vi "Version_2.0_Single_Column_Code.vi"() -> ()   [LabVIEW 2020] (continued)
                                n1984 = Subtract(x=w2419, y=w2420) -> (x-y=w2418:dbl)
                                n1985 = Absolute Value(x=w2418) -> (abs(x)=w2417:dbl)
                                }
                                frame "High Resolution Pumping" {
                                n1986 = local read "Buffer-C2 Volume \nto be Pumped"() -> (w2431:dbl)
                                n1987 = local read "Volume of Syringe"() -> (w2434:dbl)
                                n1988 = local read "Initial Plunger Position"() -> (w2438:dbl)
                                n1989 = local read "Position\nNow"() -> (w2437:dbl)
                                n1990 = Subtract(x=w2438, y=w2437) -> (x-y=w2436:dbl)
                                n1991 = Absolute Value(x=w2436) -> (abs(x)=w2435:dbl)
                                n1992 = Multiply(x=w2435, y=w2434) -> (x*y=w2433:dbl)
                                n1993 = Divide(x=w2433, y=24000.0) -> (x/y=w2430:dbl)
                                n1994 = Subtract(x=w2430, y=w2431) -> (x-y=w2429:dbl)
                                n1995 = Absolute Value(x=w2429) -> (abs(x)=w2428:dbl)
                                }
                                }
                                n1996 = local write "Buffer-C Volume\nleft to be Pumped"(w2415) -> ()
                                }
                                frame #2 {
                                n1997 = local read "Buffer-C2 Dispense\nFlow Rate (ul/min)"() -> (w2442:dbl)
                                n1998 = local read "Buffer-C2 Pumping\nResolution"() -> (w2441:T2)
                                n1999 = local read "VISA Refnum in\nfor Pump"() -> (w2444:refnum<visa-resource-name>)
                                n2000 = local read "Volume of Syringe"() -> (w2443:dbl)
                                n2001 = call "GoToAbsolutePosition(SubVI).vi"("Absolute Volume Position in Syringe (in ul)"=0.0, "Volume of Syringe"=w2443, "Resolution of Pumping"=w2441, "Flow Rate (ul/min)"=w2442, "VISA Refnum in"=w2444) -> ()  [unwired: 6 in, 1 out]
                                n2002 = local write "Suction On/Off"(FALSE ("Suction On/Off")) -> ()
                                }
                                }
                                }
                                }
                                }
                                frame #4 {
                                n2003 = local read "Stop for End of \nExperiment \nand Data Writing"() -> (w2445:bool)
                                n2004 = case shown="True" w2445 {
                                frame False {
                                }
                                frame True {
                                n2005 = local read "VISA Refnum in\nfor Pump"() -> (w2446:refnum<visa-resource-name>)
                                n2006 = call "HardStopCurrentProcess (SubVI).vi"("VISA Refnum in"=w2446) -> ()  [unwired: 11 in]
                                }
                                }
                                }
                                }
                                }
                                frame #2 {
                                # "Keeps the on-chip valve V1, V2 Open and V3 closed"
                                n2007 = while {
                                stop <- w2450 stop-if-true
                                n2008 = local read "Suction On/Off"() -> (w2451:bool)
                                n2009 = case shown="True" w2451 {
                                frame False {
                                n2010 = local read "Buffer-C2 Pumping\nResolution"() -> (w2457:T2)
                                n2011 = local read "Initial Plunger Position"() -> (w2456:dbl)
                                n2012 = local read "VISA Refnum in\nfor Pump"() -> (w2458:refnum<visa-resource-name>)
                                n2013 = local read "Position\nNow"() -> (w2454:dbl)
                                n2014 = local read "Volume of Syringe"() -> (w2455:dbl)
                                n2015 = local write "Volume being Injected \nin this process"(0.0) -> ()
                                n2016 = local write "Pause Data Collection"(FALSE) -> ()
                                n2017 = while {
                                tunnel: w2458 -> [w2465]
                                tunnel: w2457 -> [w2464]
                                tunnel: w2456 -> [w2460]
                                tunnel: w2455 -> [w2463]
                                tunnel: w2454 -> [w2459]
                                stop <- w2461 stop-if-true
                                n2018 = stacked-sequence {
                                tunnel: w2465 -> [w2471 w2493 w2518]
                                tunnel: w2464 -> [w2470 w2492 _]
                                tunnel: w2460 -> [w2468 _ _]
                                tunnel: w2463 -> [w2467 w2490 _]
                                tunnel: [_ _ w2510] -> w2461
                                tunnel: w2459 -> [_ w2488 _]
                                frame #0 {
                                # "From here on 'True Volume being injected \nin this process' represents the true total \nvolume in this process"
                                n2019 = call "AbsolutePlungerPosition (SubVI).vi"("VISA Refnum in"=w2471) -> ("Plunger Position"=w2469:i32)  [unwired: 10 in]
                                n2020 = case shown="..\"Standard Pumping\"" w2470 {
                                tunnel: w2469 -> [w2479 w2487]
                                tunnel: w2468 -> [w2478 w2486]
                                tunnel: w2467 -> [w2475 w2483]
                                tunnel: [w2472 w2480] -> w2466
                                frame .."Standard Pumping" {
                                n2021 = Subtract(x=w2479, y=w2478) -> (x-y=w2477:dbl)
                                n2022 = Absolute Value(x=w2477) -> (abs(x)=w2476:dbl)
                                n2023 = Multiply(x=w2476, y=w2475) -> (x*y=w2474:dbl)
                                n2024 = Divide(x=w2474, y=3000.0) -> (x/y=w2472:dbl)
                                }
                                frame "High Resolution Pumping".. {
                                n2025 = Subtract(x=w2487, y=w2486) -> (x-y=w2485:dbl)
                                n2026 = Absolute Value(x=w2485) -> (abs(x)=w2484:dbl)
                                n2027 = Multiply(x=w2484, y=w2483) -> (x*y=w2482:dbl)
                                n2028 = Divide(x=w2482, y=24000.0) -> (x/y=w2480:dbl)
                                }
                                }
                                n2029 = local write "True Volume being \ninjected in this\nprocess"(w2466) -> ()
                                }
                                frame #1 {
                                # "From here on 'Volume being injected \nin this process' represents the volume \nin this sub process"
                                n2030 = call "AbsolutePlungerPosition (SubVI).vi"("VISA Refnum in"=w2493) -> ("Plunger Position"=w2491:i32)  [unwired: 10 in]
                                n2031 = case shown="..\"Standard Pumping\"" w2492 {
                                tunnel: w2491 -> [w2501 w2509]
                                tunnel: w2488 -> [w2500 w2508]
                                tunnel: w2490 -> [w2497 w2505]
                                tunnel: [w2494 w2502] -> w2489
                                frame .."Standard Pumping" {
                                n2032 = Subtract(x=w2501, y=w2500) -> (x-y=w2499:dbl)
                                n2033 = Absolute Value(x=w2499) -> (abs(x)=w2498:dbl)
                                n2034 = Multiply(x=w2498, y=w2497) -> (x*y=w2496:dbl)
                                n2035 = Divide(x=w2496, y=3000.0) -> (x/y=w2494:dbl)
                                }
                                frame "High Resolution Pumping".. {
                                n2036 = Subtract(x=w2509, y=w2508) -> (x-y=w2507:dbl)
                                n2037 = Absolute Value(x=w2507) -> (abs(x)=w2506:dbl)
                                n2038 = Multiply(x=w2506, y=w2505) -> (x*y=w2504:dbl)
                                n2039 = Divide(x=w2504, y=24000.0) -> (x/y=w2502:dbl)
                                }
                                }
                                n2040 = local write "Volume being Injected \nin this process"(w2489) -> ()
                                }
                                frame #2 {
                                n2041 = local read "Stop for End of \nExperiment \nand Data Writing"() -> (w2513:bool)
                                n2042 = local read "Suction On/Off"() -> (w2514:bool)
                                n2043 = call "AbsolutePlungerPositionStatus (SubVI).vi"("VISA Refnum in"=w2518) -> ("read buffer"=w2517:string)  [unwired: 10 in]
                                n2044 = call <vilib>:"Trim Whitespace.vi"("string"=w2517) -> ("trimmed string"=w2516:string)  [unwired: 1 in]
                                n2045 = Equal?(x=w2516, y="/0`\u0003") -> (x = y?=w2512:bool)
                                n2046 = Or(x=w2514, y=w2513) -> (x .or. y?=w2511:bool)
                                n2047 = Or(x=w2512, y=w2511) -> (x .or. y?=w2510:bool)
                                }
                                }
                                n2048 = Wait (ms)(milliseconds to wait=u32 100) -> ()  [unwired: 1 out]
                                }
                                }
                                frame True {
                                n2049 = stacked-sequence {
                                frame #0 {
                                n2050 = local read "Suction Pressure\nfor EM-grid \nDeposition (mbar)"() -> (w2523:sgl)
                                n2051 = local write "Valve V4 Open"(FALSE ("Valve V4 Open")) -> ()
                                n2052 = local read "VISA Refnum in\nfor Pump"() -> (w2526:refnum<visa-resource-name>)
                                n2053 = local write "Valve V5 Open"(FALSE ("Valve V1 Open")) -> ()
                                n2054 = local write "Suction pressure \nfor grid deposition"(w2523) -> ()
                                n2055 = local write "Re-deposit Sample\nonto Grid"(FALSE ("Redeposit Sample\nonto Grid")) -> ()
                                n2056 = local write "Pause Data Collection"(TRUE ("Pause Data Collection")) -> ()
                                n2057 = call "HardStopCurrentProcess (SubVI).vi"("VISA Refnum in"=w2526) -> ()  [unwired: 11 in]
                                n2058 = local write "Valve V6 Open"(TRUE ("Valve V2 Open")) -> ()
                                n2059 = local write "Valve V7 Open"(TRUE ("Valve V3 Open")) -> ()
                                }
                                frame #1 {
                                n2060 = call <vilib>:"fgt init.vi"() -> ("error out"=w2527:errorcluster)  [unwired: 11 in]
                                n2061 = while {
                                tunnel: [w2530] -> w2528
                                tunnel: w2527 -> [w2529]
                                stop <- w2533 stop-if-true
                                # "'5' corresponds to 2nd positin in the line-up series"
                                n2062 = local read "Stop for End of \nExperiment \nand Data Writing"() -> (w2534:bool)
                                n2063 = local read "Suction Pressure\nfor EM-grid \nDeposition (mbar)"() -> (w2531:sgl)
                                n2064 = call <vilib>:"fgt set pressure.vi"("error in (no error)"=w2529, "pressure"=w2531, "pressureIndex"=u32 1) -> ("error out"=w2530:errorcluster)  [unwired: 8 in]
                                n2065 = local read "Suction On/Off"() -> (w2536:bool)
                                n2066 = Not(x=w2536) -> (.not. x?=w2535:bool)
                                n2067 = Wait (ms)(milliseconds to wait=u32 10) -> ()  [unwired: 1 out]
                                n2068 = Or(x=w2535, y=w2534) -> (x .or. y?=w2533:bool)
                                }
                                n2069 = call <vilib>:"fgt close.vi"("error in (no error)"=w2528) -> ()  [unwired: 10 in, 1 out]
                                }
                                frame #2 {
                                n2070 = call <vilib>:"fgt init.vi"() -> ("error out"=w2539:errorcluster)  [unwired: 11 in]
                                n2071 = while {
                                tunnel: w2539 -> [w2542]
                                tunnel: [w2540] -> w2538
                                stop <- w2548 stop-if-true
                                n2072 = local read "Stop for End of \nExperiment \nand Data Writing"() -> (w2544:bool)
                                n2073 = local read "Suction On/Off"() -> (w2546:bool)
                                n2074 = call <vilib>:"fgt set pressure.vi"("error in (no error)"=w2542, "pressure"=sgl 0.0, "pressureIndex"=u32 1) -> ("error out"=w2540:errorcluster)  [unwired: 8 in]
                                n2075 = Not(x=w2546) -> (.not. x?=w2545:bool)
                                n2076 = Wait (ms)(milliseconds to wait=u32 10) -> ()  [unwired: 1 out]
                                n2077 = Or(x=w2545, y=w2544) -> (x .or. y?=w2548:bool)
                                }
                                n2078 = call <vilib>:"fgt close.vi"("error in (no error)"=w2538) -> ()  [unwired: 10 in, 1 out]
                                }
                                frame #3 {
                                n2079 = local write "Valve V7 Open"(FALSE ("Valve V3 Open")) -> ()
                                n2080 = local write "Valve V5 Open"(FALSE ("Valve V1 Open")) -> ()
                                n2081 = local write "Valve V6 Open"(FALSE ("Valve V2 Open")) -> ()
                                n2082 = local write "Valve V4 Open"(FALSE ("Valve V4 Open")) -> ()
                                }
                                frame #4 {
                                n2083 = while {
                                stop <- w2554 stop-if-true
                                n2084 = local read "Stop for End of \nExperiment \nand Data Writing"() -> (w2555:bool)
                                n2085 = local read "Re-deposit Sample\nonto Grid"() -> (w2556:bool)
                                n2086 = Or(x=w2556, y=w2555) -> (x .or. y?=w2554:bool)
                                }
                                n2087 = One Button Dialog(message="Do you want to deposit sample on another grid? If yes, turn on 'Re-deposit Sample onto Grid'. Else turn on STOP ") -> ()  [unwired: 1 in, 1 out]
                                }
                                frame #5 {
                                n2088 = local write "Valve V4 Open"(TRUE ("Valve V4 Open")) -> ()
                                n2089 = local write "Valve V7 Open"(FALSE ("Valve V3 Open")) -> ()
                                n2090 = local write "Valve V5 Open"(TRUE ("Valve V1 Open")) -> ()
                                n2091 = local write "Valve V6 Open"(TRUE ("Valve V2 Open")) -> ()
                                }
                                frame #6 {
                                n2092 = local read "Re-deposit Sample\nonto Grid"() -> (w2561:bool)
                                n2093 = case shown="False" w2561 {
                                frame False {
                                n2094 = local write "Suction On/Off"(FALSE ("Suction On/Off")) -> ()
                                }
                                frame True {
                                n2095 = stacked-sequence {
                                frame #0 {
                                n2096 = local read "VISA Refnum in\nfor Pump"() -> (w2564:refnum<visa-resource-name>)
                                n2097 = call "AbsolutePlungerPosition (SubVI).vi"("VISA Refnum in"=w2564) -> ("Plunger Position"=w2563:i32)  [unwired: 10 in]
                                n2098 = local write "Position\nNow"(w2563) -> ()
                                }
                                frame #1 {
                                n2099 = local read "Buffer-C2 Pumping\nResolution"() -> (w2566:T2)
                                n2100 = case shown="\"Standard Pumping\", Default" w2566 {
                                tunnel: [w2567 w2578] -> w2565
                                frame "Standard Pumping", Default {
                                n2101 = local read "Buffer-C2 Volume \nto be Pumped"() -> (w2570:dbl)
                                n2102 = local read "Volume of Syringe"() -> (w2573:dbl)
                                n2103 = local read "Initial Plunger Position"() -> (w2577:dbl)
                                n2104 = local read "Position\nNow"() -> (w2576:dbl)
                                n2105 = Subtract(x=w2577, y=w2576) -> (x-y=w2575:dbl)
                                n2106 = Absolute Value(x=w2575) -> (abs(x)=w2574:dbl)
                                n2107 = Multiply(x=w2574, y=w2573) -> (x*y=w2572:dbl)
                                n2108 = Divide(x=w2572, y=3000.0) -> (x/y=w2569:dbl)
                                n2109 = Subtract(x=w2569, y=w2570) -> (x-y=w2568:dbl)
                                n2110 = Absolute Value(x=w2568) -> (abs(x)=w2567:dbl)
                                }
                                frame "High Resolution Pumping" {
                                n2111 = local read "Buffer-C2 Volume \nto be Pumped"() -> (w2581:dbl)
                                n2112 = local read "Volume of Syringe"() -> (w2584:dbl)
                                n2113 = local read "Initial Plunger Position"() -> (w2588:dbl)
                                n2114 = local read "Position\nNow"() -> (w2587:dbl)
                                n2115 = Subtract(x=w2588, y=w2587) -> (x-y=w2586:dbl)
                                n2116 = Absolute Value(x=w2586) -> (abs(x)=w2585:dbl)
                                n2117 = Multiply(x=w2585, y=w2584) -> (x*y=w2583:dbl)
                                n2118 = Divide(x=w2583, y=24000.0) -> (x/y=w2580:dbl)
                                n2119 = Subtract(x=w2580, y=w2581) -> (x-y=w2579:dbl)
                                n2120 = Absolute Value(x=w2579) -> (abs(x)=w2578:dbl)
                                }
                                }
                                n2121 = local write "Buffer-C Volume\nleft to be Pumped"(w2565) -> ()
                                }
                                frame #2 {
                                n2122 = local read "Buffer-C2 Dispense\nFlow Rate (ul/min)"() -> (w2592:dbl)
                                n2123 = local read "Buffer-C2 Pumping\nResolution"() -> (w2591:T2)
                                n2124 = local read "VISA Refnum in\nfor Pump"() -> (w2594:refnum<visa-resource-name>)
                                n2125 = local read "Volume of Syringe"() -> (w2593:dbl)
                                n2126 = call "GoToAbsolutePosition(SubVI).vi"("Absolute Volume Position in Syringe (in ul)"=0.0, "Volume of Syringe"=w2593, "Resolution of Pumping"=w2591, "Flow Rate (ul/min)"=w2592, "VISA Refnum in"=w2594) -> ()  [unwired: 6 in, 1 out]
                                n2127 = local write "Suction On/Off"(FALSE ("Suction On/Off")) -> ()
                                }
                                }
                                }
                                }
                                }
                                frame #7 {
                                n2128 = local read "Stop for End of \nExperiment \nand Data Writing"() -> (w2595:bool)
                                n2129 = case shown="True" w2595 {
                                frame False {
                                }
                                frame True {
                                n2130 = local read "VISA Refnum in\nfor Pump"() -> (w2596:refnum<visa-resource-name>)
                                n2131 = call "HardStopCurrentProcess (SubVI).vi"("VISA Refnum in"=w2596) -> ()  [unwired: 11 in]
                                }
                                }
                                }
                                }
                                }
                                }
                                n2132 = local read "Stop for End of \nExperiment \nand Data Writing"() -> (w2449:bool)
                                n2133 = local read "Divert Sample \nonto Grid"() -> (w2448:bool)
                                n2134 = Not(x=w2448) -> (.not. x?=w2447:bool)
                                n2135 = Or(x=w2447, y=w2449) -> (x .or. y?=w2450:bool)
                                }
                                }
                                }
                                n2136 = local write "Discard fluid \nprior to 1st \ndeposition"(TRUE ("Discard fluid \nprior to 1st \ndeposition")) -> ()
                              }
                            }
                          }
                          frame #32 {
                            n2137 = local write "Valve V2 Open"(FALSE ("Valve V2 Open")) -> ()
                            n2138 = local write "Valve V4 Open"(FALSE ("Valve V4 Open")) -> ()
                            n2139 = local write "Valve V3 Open"(FALSE ("Valve V3 Open")) -> ()
                            n2140 = local write "Valve V1 Open"(FALSE ("Valve V1 Open")) -> ()
                            n2141 = local write "Valve V6 Open"(FALSE ("Valve V6 Open")) -> ()
                            n2142 = local write "Valve V5 Open"(FALSE ("Valve V5 Open")) -> ()
                            n2143 = local write "Valve V7 Open"(FALSE ("Valve V7 Open")) -> ()
                            n2144 = local read "VISA Refnum in\nfor Valve"() -> (w2601:refnum<visa-resource-name>)
                            n2145 = local read "External Valve \nOPEN"() -> (w2600:string)
                            n2146 = Wait (ms)(milliseconds to wait=u32 500) -> ()  [unwired: 1 out]
                            n2147 = call "PortChanger_Valve (SubVI).vi"("Port Number"=w2600, "VISA Refnum in"=w2601) -> ()  [unwired: 10 in]
                          }
                          frame #33 {
                            n2148 = local read "Stopper that ends \nthe main loops"() -> (w2608:bool)
                            n2149 = Wait (ms)(milliseconds to wait=u32 500) -> ()  [unwired: 1 out]
                            n2150 = case shown="True" w2608 {
                              frame False {
                              }
                              frame True {
                                n2151 = local read "VISA Refnum in\nfor Pump"() -> (w2612:refnum<visa-resource-name>)
                                n2152 = call "HardStopCurrentProcess (SubVI).vi"("VISA Refnum in"=w2612) -> ()  [unwired: 11 in]
                              }
                            }
                            n2153 = local write "Pause Data Collection"(TRUE ("Pause Data Collection")) -> ()
                            n2154 = local write "Start the Process"(FALSE ("Start the Process")) -> ()
                            n2155 = local write "Divert Sample \nonto Grid"(FALSE ("Divert Sample \nonto Grid")) -> ()
                          }
                          frame #34 {
                            n2156 = local write "Volume being Injected \nin this process"(0.0 ("Volume being Injected \nin this process")) -> ()
                            n2157 = local write "Elution of Column-2"(FALSE ("Elution of Column-2")) -> ()
                            n2158 = local write "SEC On"(FALSE ("SEC On")) -> ()
                          }
                        }
                      }
                    }
                  }
                }
              }
              frame True {
                n2159 = local write "Pause Data Collection"(FALSE ("Pause Data Collection")) -> ()
              }
            }
          }
          frame "Automated Plunging Alone Using Purified Protein Via Chip" {
            n2160 = local read "Stopper that ends \nthe main loops"() -> (w2617:bool)
            n2161 = case shown="False" w2617 {
              frame False {
                n2162 = local read "Start the Process"() -> (w2618:bool)
                n2163 = case shown="True" w2618 {
                  frame False {
                    n2164 = local read "Stopper that ends \nthe main loops"() -> (w2620:bool)
                    n2165 = local read "Start the Process"() -> (w2619:bool)
                    n2166 = Or(x=w2620, y=w2619) -> (x .or. y?=w2621:bool)
                    n2167 = case shown="False" w2621 {
                      frame False {
                        n2168 = while {
                          stop <- w2624 stop-if-true
                          n2169 = local read "Stop for End of \nExperiment \nand Data Writing"() -> (w2623:bool)
                          n2170 = local read "Stopper that ends \nthe main loops"() -> (w2626:bool)
                          n2171 = local read "Start the Process"() -> (w2625:bool)
                          n2172 = Wait (ms)(milliseconds to wait=u32 10) -> ()  [unwired: 1 out]
                          n2173 = Or(x=w2626, y=w2625) -> (x .or. y?=w2624:bool)
                          n2174 = local write "Stopper that ends \nthe main loops"(w2623) -> ()
                        }
                        n2175 = One Button Dialog(message="Please Select the Process and Press 'Start the Process' Button") -> ()  [unwired: 1 in, 1 out]
                      }
                      frame True {
                      }
                    }
                  }
                  frame True {
                    n2176 = stacked-sequence {
                      frame #0 {
                        # "Equilibrate Column-1 with Buffer-A obtained from port-4 and pumped via port-2 and Column-2 with Buffer-C obtained from port-4 and pumped onto chip via port-6 onto the chip ...with an initial and inbetween wash of tubings while changing the buffers"
                        n2177 = stacked-sequence {
                          frame #0 {
                            n2178 = local read "VISA Refnum in\nfor Valve"() -> (w2633:refnum<visa-resource-name>)
                            n2179 = local read "External Valve \nCLOSED"() -> (w2632:string)
                            n2180 = local write "Valve V4 Open"(FALSE ("Valve V4 Open")) -> ()
                            n2181 = local write "Valve V1 Open"(FALSE ("Valve V1 Open")) -> ()
                            n2182 = local write "Valve V2 Open"(FALSE ("Valve V2 Open")) -> ()
                            n2183 = local write "Valve V3 Open"(FALSE ("Valve V3 Open")) -> ()
                            n2184 = call "PortChanger_Valve (SubVI).vi"("Port Number"=w2632, "VISA Refnum in"=w2633) -> ()  [unwired: 10 in]
                            n2185 = local write "Valve V7 Open"(FALSE ("Valve V7 Open")) -> ()
                            n2186 = local write "Valve V5 Open"(FALSE ("Valve V5 Open")) -> ()
                            n2187 = local write "Valve V6 Open"(FALSE ("Valve V6 Open")) -> ()
                            n2188 = while {
                              stop <- w2640 stop-if-true
                              # "Keeping the valve closing pressure of push pull to zero"
                              n2189 = local read "Stop for End of \nExperiment \nand Data Writing"() -> (w2641:bool)
                              n2190 = local read "Equilibriating \nColumn-1"() -> (w2642:bool)
                              n2191 = call <vilib>:"fgt set pressure.vi"("pressure"=sgl 0.0 ("order"), "pressureIndex"=1 ("module")) -> ()  [unwired: 9 in, 1 out]
                              n2192 = Or(x=w2642, y=w2641) -> (x .or. y?=w2640:bool)
                              n2193 = Wait (ms)(milliseconds to wait=u32 10) -> ()  [unwired: 1 out]
                            }
                            n2194 = local write "Equilibriating \nColumn-1"(TRUE ("Equilibriating \nColumn-1")) -> ()
                          }
                          frame #1 {
                            # "Clean the tubing with Buffer-A1"
                            n2195 = local read "N-A1"() -> (w2644:i32)
                            n2196 = for {
                              N: w2644 -> [_]
                              n2197 = stacked-sequence {
                                frame #0 {
                                n2198 = local read "VISA Refnum in\nfor Pump"() -> (w2647:refnum<visa-resource-name>)
                                n2199 = local read "Port for \nA1-Equilibriation"() -> (w2646:string)
                                n2200 = call "PortChanger (SubVI).vi"("Port Number"=w2646, "VISA Refnum in"=w2647) -> ()  [unwired: 10 in]
                                }
                                frame #1 {
                                n2201 = local read "VISA Refnum in\nfor Pump"() -> (w2648:refnum<visa-resource-name>)
                                n2202 = call "ProcessCompletionWaiter (SubVI).vi"("VISA Refnum in"=w2648) -> ()  [unwired: 11 in]
                                }
                                frame #2 {
                                n2203 = local read "VISA Refnum in\nfor Pump"() -> (w2653:refnum<visa-resource-name>)
                                n2204 = local read "Apparent Volume\nof Syringe"() -> (w2649:dbl)
                                n2205 = local read "Volume of Syringe"() -> (w2650:dbl)
                                n2206 = call "RPickUp(SubVI).vi"("Volume to be picked up"=w2649, "Volume of Syringe"=w2650, "Resolution of PickUP"=T2."Standard Pumping", "PickUp Flow Rate (ul/min)"=150.0, "VISA Refnum in"=w2653) -> ()  [unwired: 6 in, 1 out]
                                }
                                frame #3 {
                                n2207 = local read "Stopper that ends \nthe main loops"() -> (w2654:bool)
                                n2208 = local read "VISA Refnum in\nfor Pump"() -> (w2655:refnum<visa-resource-name>)
                                n2209 = case shown="True" w2654 {
                                frame False {
                                }
                                frame True {
                                n2210 = local read "VISA Refnum in\nfor Pump"() -> (w2656:refnum<visa-resource-name>)
                                n2211 = call "HardStopCurrentProcess (SubVI).vi"("VISA Refnum in"=w2656) -> ()  [unwired: 11 in]
                                }
                                }
                                n2212 = call "ProcessCompletionWaiter (SubVI).vi"("VISA Refnum in"=w2655) -> ()  [unwired: 11 in]
                                }
                                frame #4 {
                                n2213 = local read "VISA Refnum in\nfor Pump"() -> (w2658:refnum<visa-resource-name>)
                                n2214 = call "PortChanger (SubVI).vi"("Port Number"="1", "VISA Refnum in"=w2658) -> ()  [unwired: 10 in]
                                }
                                frame #5 {
                                n2215 = local read "Stopper that ends \nthe main loops"() -> (w2659:bool)
                                n2216 = local read "VISA Refnum in\nfor Pump"() -> (w2660:refnum<visa-resource-name>)
                                n2217 = case shown="True" w2659 {
                                frame False {
                                }
                                frame True {
                                n2218 = local read "VISA Refnum in\nfor Pump"() -> (w2661:refnum<visa-resource-name>)
                                n2219 = call "HardStopCurrentProcess (SubVI).vi"("VISA Refnum in"=w2661) -> ()  [unwired: 11 in]
                                }
                                }
                                n2220 = call "ProcessCompletionWaiter (SubVI).vi"("VISA Refnum in"=w2660) -> ()  [unwired: 11 in]
                                }
                                frame #6 {
                                n2221 = local read "VISA Refnum in\nfor Pump"() -> (w2666:refnum<visa-resource-name>)
                                n2222 = local read "Volume of Syringe"() -> (w2663:dbl)
                                n2223 = call "GoToAbsolutePosition(SubVI).vi"("Absolute Volume Position in Syringe (in ul)"=0.0 ("Volume to be picked up"), "Volume of Syringe"=w2663, "Resolution of Pumping"=T2."Standard Pumping" ("Resolution of PickUP"), "Flow Rate (ul/min)"=150.0 ("PickUp Flow Rate (ul/min)"), "VISA Refnum in"=w2666) -> ()  [unwired: 6 in, 1 out]
                                }
                                frame #7 {
                                n2224 = local read "Stopper that ends \nthe main loops"() -> (w2667:bool)
                                n2225 = local read "VISA Refnum in\nfor Pump"() -> (w2668:refnum<visa-resource-name>)
                                n2226 = case shown="True" w2667 {
                                frame False {
                                }
                                frame True {
                                n2227 = local read "VISA Refnum in\nfor Pump"() -> (w2669:refnum<visa-resource-name>)
                                n2228 = call "HardStopCurrentProcess (SubVI).vi"("VISA Refnum in"=w2669) -> ()  [unwired: 11 in]
                                }
                                }
                                n2229 = call "ProcessCompletionWaiter (SubVI).vi"("VISA Refnum in"=w2668) -> ()  [unwired: 11 in]
                                }
                              }
                              n2230 = local write "Pause Data Collection"(TRUE ("Pause Data Collection")) -> ()
                            }
                          }
                          frame #2 {
                            # "Switch to Port-4"
                            # "Port-4 of pump is connected to Buffer-A1"
                            n2231 = local read "Port for \nA1-Equilibriation"() -> (w2670:string)
                            n2232 = local read "VISA Refnum in\nfor Pump"() -> (w2671:refnum<visa-resource-name>)
                            n2233 = call "PortChanger (SubVI).vi"("Port Number"=w2670, "VISA Refnum in"=w2671) -> ()  [unwired: 10 in]
                          }
                          frame #3 {
                            n2234 = local read "VISA Refnum in\nfor Pump"() -> (w2672:refnum<visa-resource-name>)
                            n2235 = call "ProcessCompletionWaiter (SubVI).vi"("VISA Refnum in"=w2672) -> ()  [unwired: 11 in]
                          }
                          frame #4 {
                            n2236 = local read "VISA Refnum in\nfor Valve"() -> (w2679:refnum<visa-resource-name>)
                            n2237 = local read "External Valve \nOPEN"() -> (w2678:string)
                            n2238 = local write "Valve V3 Open"(FALSE ("Valve V3 Open")) -> ()
                            n2239 = local write "Valve V4 Open"(FALSE ("Valve V4 Open")) -> ()
                            n2240 = local write "Valve V1 Open"(TRUE ("Valve V1 Open")) -> ()
                            n2241 = local write "Valve V2 Open"(TRUE ("Valve V2 Open")) -> ()
                            n2242 = call "PortChanger_Valve (SubVI).vi"("Port Number"=w2678, "VISA Refnum in"=w2679) -> ()  [unwired: 10 in]
                            n2243 = local write "Valve V6 Open"(FALSE ("Valve V6 Open")) -> ()
                            n2244 = local write "Valve V5 Open"(FALSE ("Valve V5 Open")) -> ()
                            n2245 = local write "Valve V7 Open"(FALSE ("Valve V7 Open")) -> ()
                          }
                          frame #5 {
                            n2246 = local read "Buffer-A1 Volume \nto be  Pumped \nfor Equilibration\nof Column-1"() -> (w2685:dbl)
                            n2247 = local read "Apparent Volume\nof Syringe"() -> (w2682:dbl)
                            n2248 = Quotient & Remainder(x=w2685, y=w2682) -> (x-y*floor(x/y)=w2683:dbl, floor(x/y)=w2684:dbl)
                            n2249 = for {
                              N: w2684 -> [_]
                              n2250 = stacked-sequence {
                                frame #0 {
                                n2251 = local read "Buffer-A1 PickUp \nFlow Rate (ul/min)\nfor Equilibration \nof Column-1"() -> (w2688:dbl)
                                n2252 = local read "Buffer-A1 Pumping\nResolution \nfor Equilibration \nof Column-1"() -> (w2687:T2)
                                n2253 = local read "VISA Refnum in\nfor Pump"() -> (w2690:refnum<visa-resource-name>)
                                n2254 = local read "Apparent Volume\nof Syringe"() -> (w2686:dbl)
                                n2255 = local read "Volume of Syringe"() -> (w2689:dbl)
                                n2256 = call "RPickUp(SubVI).vi"("Volume to be picked up"=w2686, "Volume of Syringe"=w2689, "Resolution of PickUP"=w2687, "PickUp Flow Rate (ul/min)"=w2688, "VISA Refnum in"=w2690) -> ()  [unwired: 6 in, 1 out]
                                }
                                frame #1 {
                                n2257 = while {
                                stop <- w2691 stop-if-true
                                n2258 = local read "Stopper that ends \nthe main loops"() -> (w2692:bool)
                                n2259 = local read "VISA Refnum in\nfor Pump"() -> (w2693:refnum<visa-resource-name>)
                                n2260 = case shown="True" w2692 {
                                frame False {
                                }
                                frame True {
                                n2261 = local read "VISA Refnum in\nfor Pump"() -> (w2694:refnum<visa-resource-name>)
                                n2262 = call "HardStopCurrentProcess (SubVI).vi"("VISA Refnum in"=w2694) -> ()  [unwired: 11 in]
                                }
                                }
                                n2263 = call "ProcessCompletionWaiterWithOutPut (SubVI).vi"("VISA Refnum in"=w2693) -> ("Boolean"=w2691:bool)  [unwired: 10 in]
                                }
                                }
                                frame #2 {
                                # "Reads the initial Plunger Position for computing the volume dispensed"
                                n2264 = local read "VISA Refnum in\nfor Pump"() -> (w2696:refnum<visa-resource-name>)
                                n2265 = call "AbsolutePlungerPosition (SubVI).vi"("VISA Refnum in"=w2696) -> ("Plunger Position"=w2695:i32)  [unwired: 10 in]
                                n2266 = local write "Initial Plunger Position"(w2695) -> ()
                                }
                                frame #3 {
                                # "Switch to Port-2"
                                # "Port-2 of the pump is conncted to column-1 of chip"
                                n2267 = local read "VISA Refnum in\nfor Pump"() -> (w2698:refnum<visa-resource-name>)
                                n2268 = call "PortChanger (SubVI).vi"("Port Number"="2", "VISA Refnum in"=w2698) -> ()  [unwired: 10 in]
                                }
                                frame #4 {
                                n2269 = while {
                                stop <- w2699 stop-if-true
                                n2270 = local read "Stopper that ends \nthe main loops"() -> (w2700:bool)
                                n2271 = local read "VISA Refnum in\nfor Pump"() -> (w2701:refnum<visa-resource-name>)
                                n2272 = case shown="True" w2700 {
                                frame False {
                                }
                                frame True {
                                n2273 = local read "VISA Refnum in\nfor Pump"() -> (w2702:refnum<visa-resource-name>)
                                n2274 = call "HardStopCurrentProcess (SubVI).vi"("VISA Refnum in"=w2702) -> ()  [unwired: 11 in]
                                }
                                }
                                n2275 = call "ProcessCompletionWaiterWithOutPut (SubVI).vi"("VISA Refnum in"=w2701) -> ("Boolean"=w2699:bool)  [unwired: 10 in]
                                }
                                }
                                frame #5 {
                                n2276 = local read "Buffer-A1 Dispense\nFlow Rate (ul/min) \nfor Equilibration\nof Column-1"() -> (w2706:dbl)
                                n2277 = local read "Buffer-A1 Pumping\nResolution \nfor Equilibration \nof Column-1"() -> (w2705:T2)
                                n2278 = local read "VISA Refnum in\nfor Pump"() -> (w2708:refnum<visa-resource-name>)
                                n2279 = local write "Pause Data Collection"(FALSE ("Pause Data Collection")) -> ()
                                n2280 = local read "Volume of Syringe"() -> (w2707:dbl)
                                n2281 = call "GoToAbsolutePosition(SubVI).vi"("Absolute Volume Position in Syringe (in ul)"=0.0, "Volume of Syringe"=w2707, "Resolution of Pumping"=w2705, "Flow Rate (ul/min)"=w2706, "VISA Refnum in"=w2708) -> ()  [unwired: 6 in, 1 out]
                                }
                                frame #6 {
                                n2282 = local read "Buffer-A1 Pumping\nResolution \nfor Equilibration \nof Column-1"() -> (w2710:T2)
                                n2283 = local read "VISA Refnum in\nfor Pump"() -> (w2712:refnum<visa-resource-name>)
                                n2284 = local read "Initial Plunger Position"() -> (w2711:dbl)
                                n2285 = local read "Volume of Syringe"() -> (w2709:dbl)
                                n2286 = while {
                                tunnel: w2711 -> [w2719]
                                tunnel: w2712 -> [w2718]
                                tunnel: w2710 -> [w2717]
                                tunnel: w2709 -> [w2716]
                                stop <- w2714 stop-if-true
                                n2287 = stacked-sequence {
                                tunnel: w2719 -> [w2726 _]
                                tunnel: w2718 -> [w2725 w2746]
                                tunnel: w2717 -> [w2724 _]
                                tunnel: w2716 -> [w2723 _]
                                tunnel: [_ w2744] -> w2714
                                frame #0 {
                                n2288 = call "AbsolutePlungerPosition (SubVI).vi"("VISA Refnum in"=w2725) -> ("Plunger Position"=w2722:i32)  [unwired: 10 in]
                                n2289 = case shown="\"Standard Pumping\", Default" w2724 {
                                tunnel: w2726 -> [w2731 w2740]
                                tunnel: w2722 -> [w2732 w2739]
                                tunnel: [w2730 w2737] -> w2721
                                tunnel: w2723 -> [w2729 w2738]
                                frame "Standard Pumping", Default {
                                n2290 = Subtract(x=w2731, y=w2732) -> (x-y=w2728:dbl)
                                n2291 = Absolute Value(x=w2728) -> (abs(x)=w2727:dbl)
                                n2292 = Multiply(x=w2727, y=w2729) -> (x*y=w2734:dbl)
                                n2293 = Divide(x=w2734, y=3000.0) -> (x/y=w2730:dbl)
                                }
                                frame "High Resolution Pumping" {
                                n2294 = Subtract(x=w2740, y=w2739) -> (x-y=w2736:dbl)
                                n2295 = Absolute Value(x=w2736) -> (abs(x)=w2735:dbl)
                                n2296 = Multiply(x=w2735, y=w2738) -> (x*y=w2742:dbl)
                                n2297 = Divide(x=w2742, y=24000.0) -> (x/y=w2737:dbl)
                                }
                                }
                                n2298 = local write "Volume being Injected \nin this process"(w2721) -> ()
                                }
                                frame #1 {
                                n2299 = call "LSPOneStatus (SubVI).vi"("VISA Refnum in"=w2746) -> ("read buffer"=w2748:string)  [unwired: 10 in]
                                n2300 = call <vilib>:"Trim Whitespace.vi"("string"=w2748) -> ("trimmed string"=w2747:string)  [unwired: 1 in]
                                n2301 = local read "Stopper that ends \nthe main loops"() -> (w2743:bool)
                                n2302 = Equal?(x=w2747, y="/0`\u0003") -> (x = y?=w2745:bool)
                                n2303 = Or(x=w2745, y=w2743) -> (x .or. y?=w2744:bool)
                                }
                                }
                                n2304 = Wait (ms)(milliseconds to wait=u32 100) -> ()  [unwired: 1 out]
                                n2305 = local read "Stopper that ends \nthe main loops"() -> (w2713:bool)
                                n2306 = case shown="True" w2713 {
                                frame False {
                                }
                                frame True {
                                n2307 = local read "VISA Refnum in\nfor Pump"() -> (w2720:refnum<visa-resource-name>)
                                n2308 = call "HardStopCurrentProcess (SubVI).vi"("VISA Refnum in"=w2720) -> ()  [unwired: 11 in]
                                }
                                }
                                }
                                }
                                frame #7 {
                                # "Change the pump port back to Buffer-A1"
                                n2309 = local read "VISA Refnum in\nfor Pump"() -> (w2751:refnum<visa-resource-name>)
                                n2310 = local read "Port for \nA1-Equilibriation"() -> (w2750:string)
                                n2311 = local write "Pause Data Collection"(TRUE ("Pause Data Collection")) -> ()
                                n2312 = Wait (ms)(milliseconds to wait=u32 500) -> ()  [unwired: 1 out]
                                n2313 = call "PortChanger (SubVI).vi"("Port Number"=w2750, "VISA Refnum in"=w2751) -> ()  [unwired: 10 in]
                                }
                                frame #8 {
                                n2314 = local read "VISA Refnum in\nfor Pump"() -> (w2754:refnum<visa-resource-name>)
                                n2315 = local write "Volume being Injected \nin this process"(0.0 ("Volume being Injected \nin this process")) -> ()
                                n2316 = call "ProcessCompletionWaiter (SubVI).vi"("VISA Refnum in"=w2754) -> ()  [unwired: 11 in]
                                }
                              }
                            }
                            n2317 = local write "Reminder of the \nVolume to be \nPumped"(w2683) -> ()
                          }
                          frame #6 {
                            n2318 = stacked-sequence {
                              frame #0 {
                                n2319 = local read "Buffer-A1 PickUp \nFlow Rate (ul/min)\nfor Equilibration \nof Column-1"() -> (w2758:dbl)
                                n2320 = local read "Buffer-A1 Pumping\nResolution \nfor Equilibration \nof Column-1"() -> (w2757:T2)
                                n2321 = local read "VISA Refnum in\nfor Pump"() -> (w2760:refnum<visa-resource-name>)
                                n2322 = local read "Reminder of the \nVolume to be \nPumped"() -> (w2756:dbl)
                                n2323 = local read "Volume of Syringe"() -> (w2759:dbl)
                                n2324 = call "RPickUp(SubVI).vi"("Volume to be picked up"=w2756, "Volume of Syringe"=w2759, "Resolution of PickUP"=w2757, "PickUp Flow Rate (ul/min)"=w2758, "VISA Refnum in"=w2760) -> ()  [unwired: 6 in, 1 out]
                              }
                              frame #1 {
                                n2325 = while {
                                stop <- w2761 stop-if-true
                                n2326 = local read "Stopper that ends \nthe main loops"() -> (w2762:bool)
                                n2327 = local read "VISA Refnum in\nfor Pump"() -> (w2763:refnum<visa-resource-name>)
                                n2328 = case shown="True" w2762 {
                                frame False {
                                }
                                frame True {
                                n2329 = local read "VISA Refnum in\nfor Pump"() -> (w2764:refnum<visa-resource-name>)
                                n2330 = call "HardStopCurrentProcess (SubVI).vi"("VISA Refnum in"=w2764) -> ()  [unwired: 11 in]
                                }
                                }
                                n2331 = call "ProcessCompletionWaiterWithOutPut (SubVI).vi"("VISA Refnum in"=w2763) -> ("Boolean"=w2761:bool)  [unwired: 10 in]
                                }
                              }
                              frame #2 {
                                # "Reads the initial Plunger Position for computing the volume dispensed"
                                n2332 = local read "VISA Refnum in\nfor Pump"() -> (w2766:refnum<visa-resource-name>)
                                n2333 = call "AbsolutePlungerPosition (SubVI).vi"("VISA Refnum in"=w2766) -> ("Plunger Position"=w2765:i32)  [unwired: 10 in]
                                n2334 = local write "Initial Plunger Position"(w2765) -> ()
                              }
                              frame #3 {
                                # "Switch to Port-2"
                                # "Port-2 of the pump is conncted to column-1 of chip"
                                n2335 = local read "VISA Refnum in\nfor Pump"() -> (w2768:refnum<visa-resource-name>)
                                n2336 = call "PortChanger (SubVI).vi"("Port Number"="2", "VISA Refnum in"=w2768) -> ()  [unwired: 10 in]
                              }
                              frame #4 {
                                n2337 = while {
                                stop <- w2769 stop-if-true
                                n2338 = local read "Stopper that ends \nthe main loops"() -> (w2770:bool)
                                n2339 = local read "VISA Refnum in\nfor Pump"() -> (w2771:refnum<visa-resource-name>)
                                n2340 = case shown="True" w2770 {
                                frame False {
                                }
                                frame True {
                                n2341 = local read "VISA Refnum in\nfor Pump"() -> (w2772:refnum<visa-resource-name>)
                                n2342 = call "HardStopCurrentProcess (SubVI).vi"("VISA Refnum in"=w2772) -> ()  [unwired: 11 in]
                                }
                                }
                                n2343 = call "ProcessCompletionWaiterWithOutPut (SubVI).vi"("VISA Refnum in"=w2771) -> ("Boolean"=w2769:bool)  [unwired: 10 in]
                                }
                              }
                              frame #5 {
                                n2344 = local read "Buffer-A1 Pumping\nResolution \nfor Equilibration \nof Column-1"() -> (w2775:T2)
                                n2345 = local read "Buffer-A1 Dispense\nFlow Rate (ul/min) \nfor Equilibration\nof Column-1"() -> (w2776:dbl)
                                n2346 = local read "VISA Refnum in\nfor Pump"() -> (w2778:refnum<visa-resource-name>)
                                n2347 = local write "Pause Data Collection"(FALSE ("Pause Data Collection")) -> ()
                                n2348 = local read "Volume of Syringe"() -> (w2777:dbl)
                                n2349 = call "GoToAbsolutePosition(SubVI).vi"("Absolute Volume Position in Syringe (in ul)"=0.0 ("Volume to be Dispensed"), "Volume of Syringe"=w2777, "Resolution of Pumping"=w2775, "Flow Rate (ul/min)"=w2776, "VISA Refnum in"=w2778) -> ()  [unwired: 6 in, 1 out]
                              }
                              frame #6 {
                                n2350 = local read "Buffer-A1 Pumping\nResolution \nfor Equilibration \nof Column-1"() -> (w2780:T2)
                                n2351 = local read "VISA Refnum in\nfor Pump"() -> (w2782:refnum<visa-resource-name>)
                                n2352 = local read "Initial Plunger Position"() -> (w2781:dbl)
                                n2353 = local read "Volume of Syringe"() -> (w2779:dbl)
                                n2354 = while {
                                tunnel: w2781 -> [w2789]
                                tunnel: w2782 -> [w2788]
                                tunnel: w2780 -> [w2787]
                                tunnel: w2779 -> [w2786]
                                stop <- w2784 stop-if-true
                                n2355 = stacked-sequence {
                                tunnel: w2789 -> [w2796 _]
                                tunnel: w2788 -> [w2795 w2816]
                                tunnel: w2787 -> [w2794 _]
                                tunnel: w2786 -> [w2793 _]
                                tunnel: [_ w2814] -> w2784
                                frame #0 {
                                n2356 = call "AbsolutePlungerPosition (SubVI).vi"("VISA Refnum in"=w2795) -> ("Plunger Position"=w2792:i32)  [unwired: 10 in]
                                n2357 = case shown="\"Standard Pumping\", Default" w2794 {
                                tunnel: w2796 -> [w2801 w2810]
                                tunnel: w2792 -> [w2802 w2809]
                                tunnel: [w2800 w2807] -> w2791
                                tunnel: w2793 -> [w2799 w2808]
                                frame "Standard Pumping", Default {
                                n2358 = Subtract(x=w2801, y=w2802) -> (x-y=w2798:dbl)
                                n2359 = Absolute Value(x=w2798) -> (abs(x)=w2797:dbl)
                                n2360 = Multiply(x=w2797, y=w2799) -> (x*y=w2804:dbl)
                                n2361 = Divide(x=w2804, y=3000.0) -> (x/y=w2800:dbl)
                                }
                                frame "High Resolution Pumping" {
                                n2362 = Subtract(x=w2810, y=w2809) -> (x-y=w2806:dbl)
                                n2363 = Absolute Value(x=w2806) -> (abs(x)=w2805:dbl)
                                n2364 = Multiply(x=w2805, y=w2808) -> (x*y=w2812:dbl)
                                n2365 = Divide(x=w2812, y=24000.0) -> (x/y=w2807:dbl)
                                }
                                }
                                n2366 = local write "Volume being Injected \nin this process"(w2791) -> ()
                                }
                                frame #1 {
                                n2367 = call "LSPOneStatus (SubVI).vi"("VISA Refnum in"=w2816) -> ("read buffer"=w2818:string)  [unwired: 10 in]
                                n2368 = call <vilib>:"Trim Whitespace.vi"("string"=w2818) -> ("trimmed string"=w2817:string)  [unwired: 1 in]
                                n2369 = local read "Stopper that ends \nthe main loops"() -> (w2813:bool)
                                n2370 = Equal?(x=w2817, y="/0`\u0003") -> (x = y?=w2815:bool)
                                n2371 = Or(x=w2815, y=w2813) -> (x .or. y?=w2814:bool)
                                }
                                }
                                n2372 = Wait (ms)(milliseconds to wait=u32 100) -> ()  [unwired: 1 out]
                                n2373 = local read "Stopper that ends \nthe main loops"() -> (w2783:bool)
                                n2374 = case shown="True" w2783 {
                                frame False {
                                }
                                frame True {
                                n2375 = local read "VISA Refnum in\nfor Pump"() -> (w2790:refnum<visa-resource-name>)
                                n2376 = call "HardStopCurrentProcess (SubVI).vi"("VISA Refnum in"=w2790) -> ()  [unwired: 11 in]
                                }
                                }
                                }
                              }
                              frame #7 {
                                # "Change the pump port to Buffer-C1 for equilibriation of column-2"
                                n2377 = local read "VISA Refnum in\nfor Pump"() -> (w2821:refnum<visa-resource-name>)
                                n2378 = local read "Port for \nC1-Equilibriation"() -> (w2820:string)
                                n2379 = local write "Pause Data Collection"(TRUE ("Pause Data Collection")) -> ()
                                n2380 = Wait (ms)(milliseconds to wait=u32 500) -> ()  [unwired: 1 out]
                                n2381 = call "PortChanger (SubVI).vi"("Port Number"=w2820, "VISA Refnum in"=w2821) -> ()  [unwired: 10 in]
                              }
                              frame #8 {
                                n2382 = local read "VISA Refnum in\nfor Pump"() -> (w2825:refnum<visa-resource-name>)
                                n2383 = local write "Volume being Injected \nin this process"(0.0 ("Volume being Injected \nin this process")) -> ()
                                n2384 = call "ProcessCompletionWaiter (SubVI).vi"("VISA Refnum in"=w2825) -> ()  [unwired: 11 in]
                                n2385 = local write "Start the Process"(FALSE ("Start the Process")) -> ()
                              }
                            }
                          }
                          frame #7 {
                            # "Clean the tubing with Buffer-C1"
                            n2386 = local read "N-C1"() -> (w2828:i32)
                            n2387 = local write "Equilibriating \nColumn-1"(FALSE ("Equilibriating \nColumn-1")) -> ()
                            n2388 = for {
                              N: w2828 -> [_]
                              n2389 = stacked-sequence {
                                frame #0 {
                                n2390 = local read "Port for \nC1-Equilibriation"() -> (w2831:string)
                                n2391 = local read "VISA Refnum in\nfor Pump"() -> (w2832:refnum<visa-resource-name>)
                                n2392 = call "PortChanger (SubVI).vi"("Port Number"=w2831, "VISA Refnum in"=w2832) -> ()  [unwired: 10 in]
                                }
                                frame #1 {
                                n2393 = local read "VISA Refnum in\nfor Pump"() -> (w2833:refnum<visa-resource-name>)
                                n2394 = call "ProcessCompletionWaiter (SubVI).vi"("VISA Refnum in"=w2833) -> ()  [unwired: 11 in]
                                }
                                frame #2 {
                                n2395 = local read "VISA Refnum in\nfor Pump"() -> (w2838:refnum<visa-resource-name>)
                                n2396 = local read "Apparent Volume\nof Syringe"() -> (w2834:dbl)
                                n2397 = local read "Volume of Syringe"() -> (w2835:dbl)
                                n2398 = call "RPickUp(SubVI).vi"("Volume to be picked up"=w2834, "Volume of Syringe"=w2835, "Resolution of PickUP"=T2."Standard Pumping", "PickUp Flow Rate (ul/min)"=150.0, "VISA Refnum in"=w2838) -> ()  [unwired: 6 in, 1 out]
                                }
                                frame #3 {
                                n2399 = local read "Stopper that ends \nthe main loops"() -> (w2839:bool)
                                n2400 = local read "VISA Refnum in\nfor Pump"() -> (w2840:refnum<visa-resource-name>)
                                n2401 = case shown="True" w2839 {
                                frame False {
                                }
                                frame True {
                                n2402 = local read "VISA Refnum in\nfor Pump"() -> (w2841:refnum<visa-resource-name>)
                                n2403 = call "HardStopCurrentProcess (SubVI).vi"("VISA Refnum in"=w2841) -> ()  [unwired: 11 in]
                                }
                                }
                                n2404 = call "ProcessCompletionWaiter (SubVI).vi"("VISA Refnum in"=w2840) -> ()  [unwired: 11 in]
                                }
                                frame #4 {
                                n2405 = local read "VISA Refnum in\nfor Pump"() -> (w2843:refnum<visa-resource-name>)
                                n2406 = call "PortChanger (SubVI).vi"("Port Number"="1", "VISA Refnum in"=w2843) -> ()  [unwired: 10 in]
                                }
                                frame #5 {
                                n2407 = local read "Stopper that ends \nthe main loops"() -> (w2844:bool)
                                n2408 = local read "VISA Refnum in\nfor Pump"() -> (w2845:refnum<visa-resource-name>)
                                n2409 = case shown="True" w2844 {
                                frame False {
                                }
                                frame True {
                                n2410 = local read "VISA Refnum in\nfor Pump"() -> (w2846:refnum<visa-resource-name>)
                                n2411 = call "HardStopCurrentProcess (SubVI).vi"("VISA Refnum in"=w2846) -> ()  [unwired: 11 in]
                                }
                                }
                                n2412 = call "ProcessCompletionWaiter (SubVI).vi"("VISA Refnum in"=w2845) -> ()  [unwired: 11 in]
                                }
                                frame #6 {
                                n2413 = local read "VISA Refnum in\nfor Pump"() -> (w2851:refnum<visa-resource-name>)
                                n2414 = local read "Volume of Syringe"() -> (w2848:dbl)
                                n2415 = call "GoToAbsolutePosition(SubVI).vi"("Absolute Volume Position in Syringe (in ul)"=0.0 ("Volume to be picked up"), "Volume of Syringe"=w2848, "Resolution of Pumping"=T2."Standard Pumping" ("Resolution of PickUP"), "Flow Rate (ul/min)"=150.0 ("PickUp Flow Rate (ul/min)"), "VISA Refnum in"=w2851) -> ()  [unwired: 6 in, 1 out]
                                }
                                frame #7 {
                                n2416 = local read "Stopper that ends \nthe main loops"() -> (w2852:bool)
                                n2417 = local read "VISA Refnum in\nfor Pump"() -> (w2853:refnum<visa-resource-name>)
                                n2418 = case shown="True" w2852 {
                                frame False {
                                }
                                frame True {
                                n2419 = local read "VISA Refnum in\nfor Pump"() -> (w2854:refnum<visa-resource-name>)
                                n2420 = call "HardStopCurrentProcess (SubVI).vi"("VISA Refnum in"=w2854) -> ()  [unwired: 11 in]
                                }
                                }
                                n2421 = call "ProcessCompletionWaiter (SubVI).vi"("VISA Refnum in"=w2853) -> ()  [unwired: 11 in]
                                }
                              }
                            }
                            n2422 = local write "Pause Data Collection"(TRUE ("Pause Data Collection")) -> ()
                            n2423 = local write "Equilibriating \nColumn-2"(TRUE ("Equilibriating \nColumn-2")) -> ()
                          }
                          frame #8 {
                            n2424 = local read "Buffer-C1 Volume \nto be  Pumped \nfor Equilibration\nof Column-2"() -> (w2858:dbl)
                            n2425 = local read "Apparent Volume\nof Syringe"() -> (w2855:dbl)
                            n2426 = Quotient & Remainder(x=w2858, y=w2855) -> (x-y*floor(x/y)=w2856:dbl, floor(x/y)=w2857:dbl)
                            n2427 = for {
                              N: w2857 -> [_]
                              n2428 = stacked-sequence {
                                frame #0 {
                                n2429 = local read "VISA Refnum in\nfor Pump"() -> (w2860:refnum<visa-resource-name>)
                                n2430 = local read "Port for \nC1-Equilibriation"() -> (w2859:string)
                                n2431 = call "PortChanger (SubVI).vi"("Port Number"=w2859, "VISA Refnum in"=w2860) -> ()  [unwired: 10 in]
                                }
                                frame #1 {
                                n2432 = local read "VISA Refnum in\nfor Pump"() -> (w2861:refnum<visa-resource-name>)
                                n2433 = call "ProcessCompletionWaiter (SubVI).vi"("VISA Refnum in"=w2861) -> ()  [unwired: 11 in]
                                }
                                frame #2 {
                                n2434 = local read "Buffer-C1 PickUp \nFlow Rate (ul/min)\nfor Equilibration \nof Column-2"() -> (w2864:dbl)
                                n2435 = local read "Buffer-C1 Pumping\nResolution \nfor Equilibration \nof Column-2"() -> (w2863:T2)
                                n2436 = local read "VISA Refnum in\nfor Pump"() -> (w2866:refnum<visa-resource-name>)
                                n2437 = local read "Apparent Volume\nof Syringe"() -> (w2862:dbl)
                                n2438 = local read "Volume of Syringe"() -> (w2865:dbl)
                                n2439 = call "RPickUp(SubVI).vi"("Volume to be picked up"=w2862, "Volume of Syringe"=w2865, "Resolution of PickUP"=w2863, "PickUp Flow Rate (ul/min)"=w2864, "VISA Refnum in"=w2866) -> ()  [unwired: 6 in, 1 out]
                                }
                                frame #3 {
                                n2440 = while {
                                stop <- w2867 stop-if-true
                                n2441 = local read "Stopper that ends \nthe main loops"() -> (w2868:bool)
                                n2442 = local read "VISA Refnum in\nfor Pump"() -> (w2869:refnum<visa-resource-name>)
                                n2443 = case shown="True" w2868 {
                                frame False {
                                }
                                frame True {
                                n2444 = local read "VISA Refnum in\nfor Pump"() -> (w2870:refnum<visa-resource-name>)
                                n2445 = call "HardStopCurrentProcess (SubVI).vi"("VISA Refnum in"=w2870) -> ()  [unwired: 11 in]
                                }
                                }
                                n2446 = call "ProcessCompletionWaiterWithOutPut (SubVI).vi"("VISA Refnum in"=w2869) -> ("Boolean"=w2867:bool)  [unwired: 10 in]
                                }
                                }
                                frame #4 {
                                # "Reads the initial Plunger Position for computing the volume dispensed"
                                n2447 = local read "VISA Refnum in\nfor Pump"() -> (w2872:refnum<visa-resource-name>)
                                n2448 = call "AbsolutePlungerPosition (SubVI).vi"("VISA Refnum in"=w2872) -> ("Plunger Position"=w2871:i32)  [unwired: 10 in]
                                n2449 = local write "Initial Plunger Position"(w2871) -> ()
                                }
                                frame #5 {
                                # "Switch to Port-10"
                                # "Port-10 of the pump is conncted to column-2 of chip"
                                n2450 = local read "VISA Refnum in\nfor Pump"() -> (w2874:refnum<visa-resource-name>)
                                n2451 = call "PortChanger (SubVI).vi"("Port Number"="10", "VISA Refnum in"=w2874) -> ()  [unwired: 10 in]
                                }
                                frame #6 {
                                n2452 = while {
                                stop <- w2875 stop-if-true
                                n2453 = local read "Stopper that ends \nthe main loops"() -> (w2876:bool)
                                n2454 = local read "VISA Refnum in\nfor Pump"() -> (w2877:refnum<visa-resource-name>)
                                n2455 = case shown="True" w2876 {
                                frame False {
                                }
                                frame True {
                                n2456 = local read "VISA Refnum in\nfor Pump"() -> (w2878:refnum<visa-resource-name>)
                                n2457 = call "HardStopCurrentProcess (SubVI).vi"("VISA Refnum in"=w2878) -> ()  [unwired: 11 in]
                                }
                                }
                                n2458 = call "ProcessCompletionWaiterWithOutPut (SubVI).vi"("VISA Refnum in"=w2877) -> ("Boolean"=w2875:bool)  [unwired: 10 in]
                                }
                                }
                                frame #7 {
                                # "Buffer-C pumped for column non-interference"
                                # "Keeps the AMF valve after column-1 open and valve after column-2 closed"
                                n2459 = local read "Buffer-C1 Dispense\nFlow Rate (ul/min) \nfor Equilibration\nof Column-2"() -> (w2891:dbl)
                                n2460 = local read "Buffer-C1 Pumping\nResolution \nfor Equilibration \nof Column-2"() -> (w2890:T2)
                                n2461 = local read "VISA Refnum in\nfor Pump"() -> (w2893:refnum<visa-resource-name>)
                                n2462 = local write "Pause Data Collection"(FALSE ("Pause Data Collection")) -> ()
                                n2463 = local read "Volume of Syringe"() -> (w2892:dbl)
                                n2464 = call "GoToAbsolutePosition(SubVI).vi"("Absolute Volume Position in Syringe (in ul)"=0.0, "Volume of Syringe"=w2892, "Resolution of Pumping"=w2890, "Flow Rate (ul/min)"=w2891, "VISA Refnum in"=w2893) -> ()  [unwired: 6 in, 1 out]
                                n2465 = local write "Valve V1 Open"(FALSE ("Valve V1 Open")) -> ()
                                n2466 = local write "Valve V2 Open"(TRUE ("Valve V2 Open")) -> ()
                                n2467 = local write "Valve V4 Open"(FALSE ("Valve V4 Open")) -> ()
                                n2468 = local write "Valve V3 Open"(TRUE ("Valve V3 Open")) -> ()
                                n2469 = local read "VISA Refnum in\nfor Valve"() -> (w2884:refnum<visa-resource-name>)
                                n2470 = local read "External Valve \nOPEN"() -> (w2883:string)
                                n2471 = local write "Valve V5 Open"(FALSE ("Valve V5 Open")) -> ()
                                n2472 = local write "Valve V6 Open"(FALSE ("Valve V6 Open")) -> ()
                                n2473 = local write "Valve V7 Open"(FALSE ("Valve V7 Open")) -> ()
                                n2474 = call "PortChanger_Valve (SubVI).vi"("Port Number"=w2883, "VISA Refnum in"=w2884) -> ()  [unwired: 10 in]
                                }
                                frame #8 {
                                n2475 = local read "Buffer-C1 Pumping\nResolution \nfor Equilibration \nof Column-2"() -> (w2895:T2)
                                n2476 = local read "VISA Refnum in\nfor Pump"() -> (w2897:refnum<visa-resource-name>)
                                n2477 = local read "Initial Plunger Position"() -> (w2896:dbl)
                                n2478 = local read "Volume of Syringe"() -> (w2894:dbl)
                                n2479 = while {
                                tunnel: w2896 -> [w2904]
                                tunnel: w2897 -> [w2903]
                                tunnel: w2895 -> [w2902]
                                tunnel: w2894 -> [w2901]
                                stop <- w2899 stop-if-true
                                n2480 = stacked-sequence {
                                tunnel: w2904 -> [w2911 _]
                                tunnel: w2903 -> [w2910 w2935]
                                tunnel: w2902 -> [w2909 _]
                                tunnel: w2901 -> [w2908 _]
                                tunnel: [_ w2933] -> w2899
                                frame #0 {
                                n2481 = call "AbsolutePlungerPosition (SubVI).vi"("VISA Refnum in"=w2910) -> ("Plunger Position"=w2907:i32)  [unwired: 10 in]
                                n2482 = case shown="\"Standard Pumping\", Default" w2909 {
                                tunnel: w2911 -> [w2916 w2925]
                                tunnel: w2907 -> [w2917 w2924]
                                tunnel: [w2915 w2922] -> w2906
                                tunnel: w2908 -> [w2914 w2923]
                                frame "Standard Pumping", Default {
                                n2483 = Subtract(x=w2916, y=w2917) -> (x-y=w2913:dbl)
                                n2484 = Absolute Value(x=w2913) -> (abs(x)=w2912:dbl)
                                n2485 = Multiply(x=w2912, y=w2914) -> (x*y=w2919:dbl)
                                n2486 = Divide(x=w2919, y=3000.0) -> (x/y=w2915:dbl)
                                }
                                frame "High Resolution Pumping" {
                                n2487 = Subtract(x=w2925, y=w2924) -> (x-y=w2921:dbl)
                                n2488 = Absolute Value(x=w2921) -> (abs(x)=w2920:dbl)
                                n2489 = Multiply(x=w2920, y=w2923) -> (x*y=w2927:dbl)
                                n2490 = Divide(x=w2927, y=24000.0) -> (x/y=w2922:dbl)
                                }
                                }
                                n2491 = local write "Volume being Injected \nin this process"(w2906) -> ()
                                }
                                frame #1 {
                                n2492 = local read "Buffer-C Volume \nto be Pumped for\nColumn \nnon-interference"() -> (w2931:dbl)
                                n2493 = local read "Volume being Injected \nin this process"() -> (w2932:dbl)
                                n2494 = local read "Stopper that ends \nthe main loops"() -> (w2930:bool)
                                n2495 = call "LSPOneStatus (SubVI).vi"("VISA Refnum in"=w2935) -> ("read buffer"=w2937:string)  [unwired: 10 in]
                                n2496 = call <vilib>:"Trim Whitespace.vi"("string"=w2937) -> ("trimmed string"=w2936:string)  [unwired: 1 in]
                                n2497 = Equal?(x=w2936, y="/0`\u0003") -> (x = y?=w2934:bool)
                                n2498 = Greater Or Equal?(x=w2932, y=w2931) -> (x >= y?=w2929:bool)
                                n2499 = Or(x=w2930, y=w2929) -> (x .or. y?=w2928:bool)
                                n2500 = Or(x=w2934, y=w2928) -> (x .or. y?=w2933:bool)
                                }
                                }
                                n2501 = Wait (ms)(milliseconds to wait=u32 100) -> ()  [unwired: 1 out]
                                n2502 = local read "Stopper that ends \nthe main loops"() -> (w2898:bool)
                                n2503 = case shown="True" w2898 {
                                frame False {
                                }
                                frame True {
                                n2504 = local read "VISA Refnum in\nfor Pump"() -> (w2905:refnum<visa-resource-name>)
                                n2505 = call "HardStopCurrentProcess (SubVI).vi"("VISA Refnum in"=w2905) -> ()  [unwired: 11 in]
                                }
                                }
                                }
                                }
                                frame #9 {
                                # "Keeps the AMF valve after column-1 closed and valve after column-2 open"
                                n2506 = local read "VISA Refnum in\nfor Valve"() -> (w2943:refnum<visa-resource-name>)
                                n2507 = local read "External Valve \nCLOSED"() -> (w2942:string)
                                n2508 = local write "Valve V3 Open"(FALSE ("Valve V3 Open")) -> ()
                                n2509 = local write "Valve V2 Open"(FALSE ("Valve V2 Open")) -> ()
                                n2510 = local write "Valve V4 Open"(TRUE ("Valve V1 Open")) -> ()
                                n2511 = local write "Valve V1 Open"(FALSE ("Valve V1 Open")) -> ()
                                n2512 = call "PortChanger_Valve (SubVI).vi"("Port Number"=w2942, "VISA Refnum in"=w2943) -> ()  [unwired: 10 in]
                                n2513 = local write "Valve V5 Open"(TRUE ("Valve V4 Open")) -> ()
                                n2514 = local write "Valve V7 Open"(TRUE ("Valve V6 Open")) -> ()
                                n2515 = local write "Valve V6 Open"(FALSE ("Valve V6 Open")) -> ()
                                }
                                frame #10 {
                                n2516 = local read "Buffer-C1 Pumping\nResolution \nfor Equilibration \nof Column-2"() -> (w2949:T2)
                                n2517 = local read "VISA Refnum in\nfor Pump"() -> (w2951:refnum<visa-resource-name>)
                                n2518 = local read "Initial Plunger Position"() -> (w2950:dbl)
                                n2519 = local read "Volume of Syringe"() -> (w2948:dbl)
                                n2520 = while {
                                tunnel: w2950 -> [w2958]
                                tunnel: w2951 -> [w2957]
                                tunnel: w2949 -> [w2956]
                                tunnel: w2948 -> [w2955]
                                stop <- w2953 stop-if-true
                                n2521 = stacked-sequence {
                                tunnel: w2958 -> [w2965 _]
                                tunnel: w2957 -> [w2964 w2985]
                                tunnel: w2956 -> [w2963 _]
                                tunnel: w2955 -> [w2962 _]
                                tunnel: [_ w2983] -> w2953
                                frame #0 {
                                n2522 = call "AbsolutePlungerPosition (SubVI).vi"("VISA Refnum in"=w2964) -> ("Plunger Position"=w2961:i32)  [unwired: 10 in]
